vi "testWrongControlName.vi"() -> ()   [LabVIEW 2019, in "TestCaseTest.lvlib" / "Theory.lvlib"]
uses:
  Theory.lvlib
  TestCase/Theory/Theory.lvclass
  TestCaseTestSupport/FakeTheory.vi
  TestCaseTestSupport/TestCaseTestSupport.lvlib
  Assertion/Assertion.lvlib
panel:
  out "error out":errorcluster
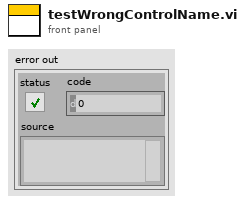
[diagram p1: front panel]
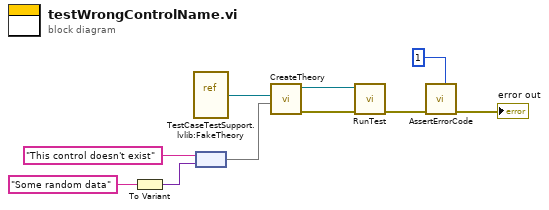
[diagram p0: block diagram]
diagram:
  n1 = To Variant(anything="Some random data" ("key")) -> (Variant=w3:variant)
  n2 = vi-ref "TestCaseTestSupport.lvlib:FakeTheory.vi"() -> (w1:refnum<vi>)
  n3 = node("This control doesn't exist" ("key"), w3) -> (w4:map{string, variant})
  n4 = call "CreateTheory.vi"("Control Data"=w4, "VI Refnum"=w1) -> ("error out"=w9:errorcluster, "Theory"=w10:refnum<class "Theory.lvclass">)  [unwired: 8 in]
  n5 = call-dynamic "RunTest.vi"("error in (no error)"=w9, "Theory in"=w10) -> ("error out"=w8:errorcluster)  [unwired: 8 in, 1 out]
  n6 = call "AssertErrorCode.vi"("Expected"=1, "error in (no error)"=w8) -> ("error out"=→"error out":errorcluster)  [unwired: 9 in]
